vi "Sensor Board Example LaunchPad.vi"() -> ()   [LabVIEW 2011]
panel:
  out "VCC":dbl(slide) scale=0.0..2.5 scale format="%.2f"
  out "Temp":dbl(slide) scale=0.0..2.5 scale format="%.2f"
  out "P1.7":dbl(slide) scale=0.0..2.5 scale format="%.2f"
  out "P1.6":dbl(slide) scale=0.0..2.5 scale format="%.2f"
  out "P1.5":dbl(slide) scale=0.0..2.5 scale format="%.2f"
  out "P1.4":dbl(slide) scale=0.0..2.5 scale format="%.2g"
  out "P1.0":dbl(slide) scale=0.0..2.5 scale format="%.2f"
  in  "stop":bool
  out "CurrentPath":path
  out "new picture":picture
  # "Launchpad Sensor Booster Pack \n                                with LILPv3"
  # "0"
  # "4"
  # "x"
  # "y"
  # "z"
  # "T"
  # "V"
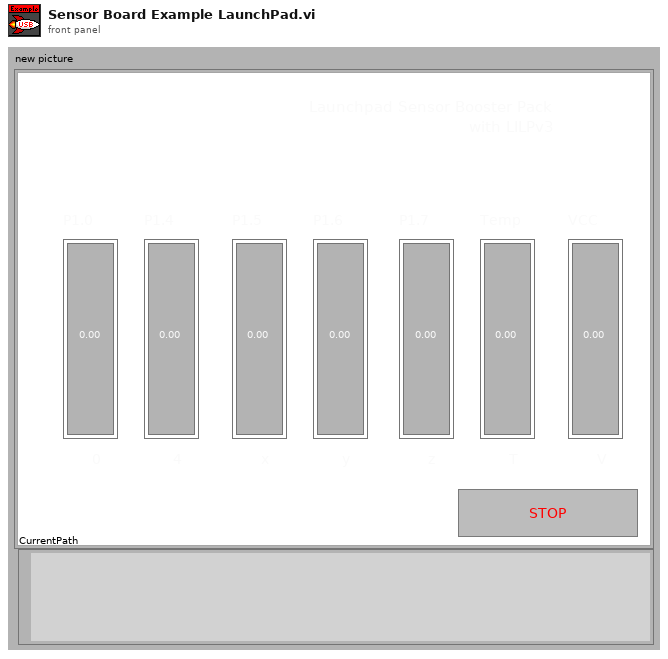
[diagram p1: front panel]
types:
  T1 = typedef "imagedata.ctl" = cluster{"image type":i32, "image depth":i32, "image":u8[], "mask":u8[], "colors":u32[], "Rectangle":cluster{"left":i16, "top":i16, "right":i16, "bottom":i16}}
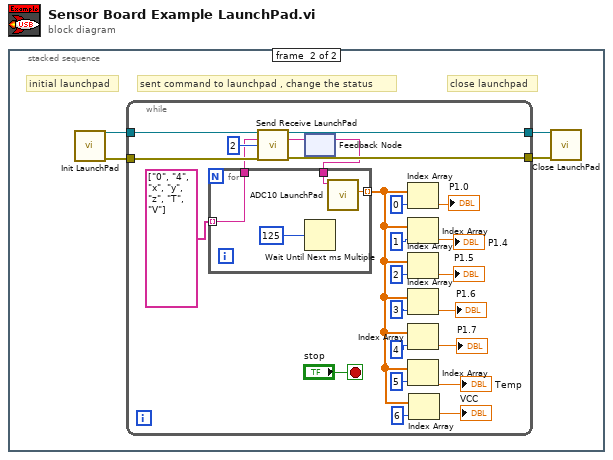
[diagram p0: block diagram]
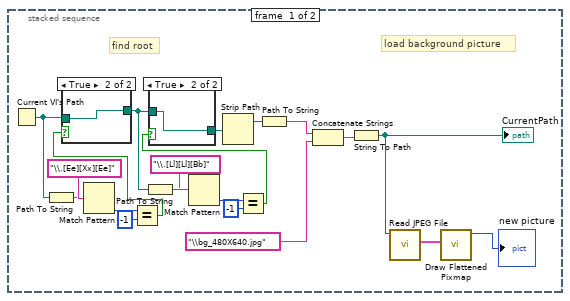
[diagram p2: hidden frame]
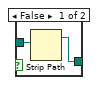
[diagram p3: hidden frame]
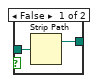
[diagram p4: hidden frame]
diagram:
  n1 = stacked-sequence {
    frame #0 {
      # "load background picture"
      # "find root"
      n2 = Current VI's Path() -> (path=w9:path)
      n3 = Path To String(path=w9) -> (string=w8:string)
      n4 = Match Pattern(string=w8, regular expression="\\.[Ee][Xx][Ee]") -> (offset past match=w6:i32)  [unwired: 1 in, 3 out]
      n5 = Equal?(x=w6, y=-1) -> (x = y?=w18:bool)
      n6 = case shown="True" w18 {
        tunnel: [w24 w26] -> w15
        tunnel: w9 -> [w25 w26]
        frame False {
          n7 = Strip Path(path=w25) -> (stripped path=w24:path)  [unwired: 1 out]
        }
        frame True {
        }
      }
      n8 = Path To String(path=w15) -> (string=w12:string)
      n9 = Match Pattern(string=w12, regular expression="\\.[Ll][Ll][Bb]") -> (offset past match=w14:i32)  [unwired: 1 in, 3 out]
      n10 = Equal?(x=w14, y=-1) -> (x = y?=w17:bool)
      n11 = case shown="True" w17 {
        tunnel: [w21 w23] -> w16
        tunnel: w15 -> [w22 w23]
        frame False {
          n12 = Strip Path(path=w22) -> (stripped path=w21:path)  [unwired: 1 out]
        }
        frame True {
        }
      }
      n13 = Strip Path(path=w16) -> (stripped path=w5:path)  [unwired: 1 out]
      n14 = Path To String(path=w5) -> (string=w2:string)
      n15 = Concatenate Strings(w2, "\\bg_480X640.jpg") -> (w3:string)
      n16 = String To Path(string=w3) -> (path=w1:path)
      "CurrentPath" <- w1
      n17 = call <vilib>:"Read JPEG File.vi"("path to JPEG file"=w1) -> ("image data"=w19:T1)  [unwired: 8 in, 2 out]
      n18 = call <vilib>:"Draw Flattened Pixmap.vi"("image data"=w19) -> ("new picture"=→"new picture":picture)  [unwired: 8 in]
    }
    frame #1 {
      # "close launchpad"
      # "sent command to launchpad , change the status"
      # "initial launchpad"
      n19 = call "Init LaunchPad.vi"() -> ("error out"=w27:errorcluster, "VISA resource name out"=w30:refnum<visa-resource-name>)  [unwired: 10 in]
      n20 = while {
        tunnel: w30 -> [w55]
        tunnel: [w54] -> w29
        tunnel: [w53] -> w28
        tunnel: w27 -> [w52]
        stop <- "stop" stop-if-true
        n21 = feedback #1() -> (w31:string)  [unwired: 1 in]
        n22 = for {
          tunnel: string[] ["0", "4", "x", "y", "z", "T", "V"] -> [w59] mode=indexing
          tunnel: [w59] -> w48
          tunnel: w31 -> [w58]
          tunnel: [w57] -> w35 mode=indexing
          n23 = Wait Until Next ms Multiple(millisecond multiple=u32 125) -> ()  [unwired: 1 out]
          n24 = call "ADC10 LaunchPad.vi"("string"=w58) -> ("ADC10 (Volt)"=w57:dbl)  [unwired: 9 in, 1 out]
        }
        n25 = call "Send Receive LaunchPad.vi"("VISA resource"=w55, "write buffer"=w48, "Bytes To Read (0)"=u8 2, "error in"=w52) -> ("VISA resource 2"=w54:refnum<visa-resource-name>, "Read Buffer"=w32:string, "error out"=w53:errorcluster)  [unwired: 9 in]
        n26 = feedback-in #1(w32) -> ()
        n27 = Index Array(array=w35, index=0) -> (element=→"P1.0":dbl)
        n28 = Index Array(array=w35, index=1) -> (element=→"P1.4":dbl)
        n29 = Index Array(array=w35, index=2) -> (element=→"P1.5":dbl)
        n30 = Index Array(array=w35, index=3) -> (element=→"P1.6":dbl)
        n31 = Index Array(array=w35, index=4) -> (element=→"P1.7":dbl)
        n32 = Index Array(array=w35, index=5) -> (element=→"Temp":dbl)
        n33 = Index Array(array=w35, index=6) -> (element=→"VCC":dbl)
      }
      n34 = call "Close LaunchPad.vi"("VISA resource name"=w29, "error in"=w28) -> ()  [unwired: 13 in, 1 out]
    }
  }
